vi "Shooter Ready.vi"() -> ()   [LabVIEW 2011]
panel:
  in  "Shooter Ready":bool
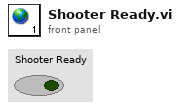
[diagram p1: front panel]
diagram:
